vi "Build Report.vi"(8 "error in (no error)":errorcluster, 11 "Sequencer Module runtime in":refnum<class "Sequencer Module runtime.lvclass">) -> (0 "error out":errorcluster, 3 "Sequencer Module runtime out":refnum<class "Sequencer Module runtime.lvclass">)   [LabVIEW 2015, in "Sequencer Module runtime.lvclass"]
uses:
  Sequencer Module runtime.lvclass
  Sequencer Module runtime.lvclass/Sequencer Module runtime.ctl
  classes/Results List/Results List.lvclass
  classes/Result/Result.lvclass
  classes/Sequence/Execution/Sequence.lvclass
  classes/Result Processor/Execution/ResultProcessor.lvclass
panel:
  out "Array":string[][](array[string])
  in  "index":i32
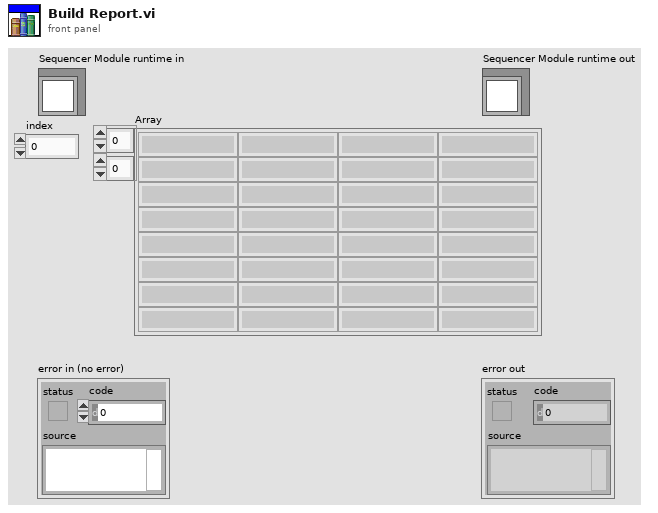
[diagram p1: front panel]
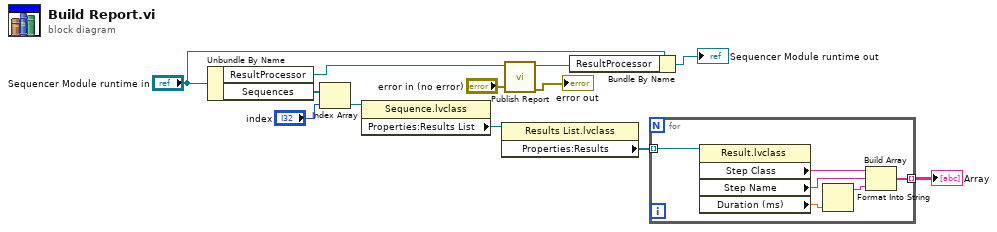
[diagram p0: block diagram]
diagram:
  n1 = Unbundle By Name("Sequencer Module runtime in") -> ("ResultProcessor"=w4:refnum<class "ResultProcessor.lvclass">, "Sequences"=w12:refnum<class "Sequence.lvclass">[])
  n2 = Index Array(array=w12, index="index") -> (element=w10:refnum<class "Sequence.lvclass">)
  n3 = property class="Sequence.lvclass"(reference=w10) -> ("Properties:Results List"=w9:refnum<class "Results List.lvclass">)  [unwired: 1 in, 2 out]
  n4 = property class="Results List.lvclass"(reference=w9) -> ("Properties:Results"=w8:refnum<class "Result.lvclass">[])  [unwired: 1 in, 2 out]
  n5 = call "Publish Report.vi"("error in (no error)"="error in (no error)", "ResultProcessor in"=w4) -> ("error out"=→"error out":errorcluster, "ResultProcessor out"=w3:refnum<class "ResultProcessor.lvclass">)  [unwired: 8 in]
  n6 = Bundle By Name(cluster="Sequencer Module runtime in", "ResultProcessor"=w3) -> (→"Sequencer Module runtime out":refnum<class "Sequencer Module runtime.lvclass">)
  n7 = for {
    tunnel: w8 -> [w18] mode=indexing
    tunnel: [w15] -> w7 mode=indexing
    n8 = property class="Result.lvclass"(reference=w18) -> ("Step Class"=w17:string, "Step Name"=w16:string, "Duration (ms)"=w14:dbl)  [unwired: 1 in, 2 out]
    n9 = Format Into String(w14) -> (resulting string=w13:string)  [unwired: 3 in, 1 out]
    n10 = Build Array(w17, w16, w13) -> (w15:string[])
  }
  "Array" <- w7
